vi "Camera Barcode.vi"() -> ()   [LabVIEW 2017]
uses:
  IMAQCV/PIIO/Core/PIIO DIO.ctl
  IMAQCV/GPIO/GPIO Pins.ctl
  <vilib>/Platform/TimedLoop/XDataNode/timing_clust.ctl
  <vilib>/Platform/TimedLoop/XDataNode/nitl_modes.ctl
  <vilib>/Platform/TimedLoop/XDataNode/wakeup.ctl
  <vilib>/vision/Instrument.llb/Barcode Search Options.ctl
  <vilib>/platform/TimedLoop/XDataNode/XDataNode.xnode
  IMAQCV/PIIO.lvlib
  IMAQCV/IMAQCV.lvlib
  IMAQCV/LVOpenCV.lvlib
  <vilib>/Platform/TimedLoop/XDataNode/XDNodeRunTimeDep.lvlib
  <vilib>/vision/NI_Vision_Development_Module.lvlib
panel:
  in  "PIN":T1 items=["L1", "L2"]
  in  "Shutter (us, 0=auto)":i32
  in  "Effect":T2(ring)
  in  "Meter":enum16{"AVERAGE", "SPOT", "BACKLIT", "MATRIX"}(ring)
  in  "AWB":T3(ring)
  in  "Flip Vertical":bool
  in  "Flip Horizontal":bool
  in  "Rotation":u16(ring) items=["0", "90", "180", "270"]
  in  "Sharpness":i32(slide)=50 scale=0.0..100.0
  in  "Saturation":i32(slide)=50 scale=0.0..100.0
  in  "Contrast":i32(slide)=50 scale=0.0..100.0
  in  "Brightness":i32(slide)=50 scale=0.0..100.0
  in  "Gain (0=auto)":i32(slide) scale=0.0..100.0
  in  "LED Control":bool
  in  "FPS":i32=90
  in  "RGB LED 8x8":u32[][](array[colorbox])=[[0, 0, 16777215, 16777215, 16777215, 16777215, 16777215, 16777215], [0, 16777215, 16777215, 16777215, 16777215, 16777215, 16777215, 16777215], [16777215, 16777215, 16777215, 16777215, 16777215, 16777215, 16777215, 16777215], [16777215, 16777215, 0, 0, 0, 0, 0, 0], [16777215, 16777215, 0, 0, 0, 0, 0, 0], [16777215, 16777215, 0, 0, 0, 0, 0, 0], [16777215, 16777215, 0, 0, 0, 0, 0, 0], [0, 16777215, 16777215, 16777215, 16777215, 0, 0, 0]]
  out "picture":picture
  in  "Image Size":T4(ring)=enum."640 (H)   x  480 (V) "
  in  "LED Flash":bool
  out "moving speed (ms)":u32
  out "barcode process time (ms)":u32
  out "Barcode ANSI/CEN/ISO Grading Report":T5(array[cluster])
  out "Barcode Read":cluster{"Data":string, "Barcode Type":string}[](array[cluster])
  out "Number of Barcodes Found":u32
  in  "delay (ms)":u32=150
  out "DI-CH4":bool
  out "DI-CH3":bool
  out "DI-CH2":bool
  out "DI-CH1":bool
  in  "stop":bool
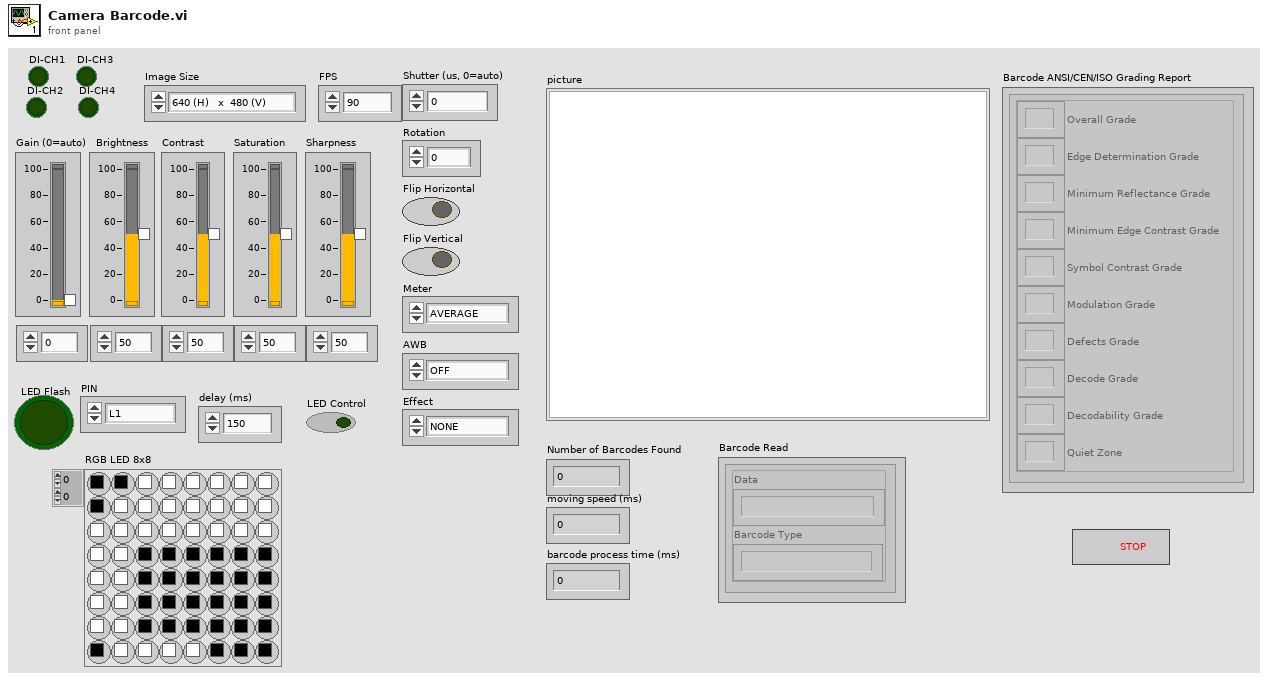
[diagram p1: front panel]
types:
  T1 = typedef "PIIO.lvlib/PIIO DIO.ctl" = u8
  T2 = enum16{"NONE", "NEGATIVE", "SOLARIZE", "SKETCH", "DENOISE", "EMBOSS", "OILPAINT", "HATCH", "GPEN", "PASTEL", "WATERCOLOR", "FILM", "BLUR", "SATURATION", "COLORSWAP", "WASHEDOUT", "POSTERISE", "COLORPOINT", "COLORBALANCE", "CARTOON"}
  T3 = enum16{"OFF", "AUTO", "SUNLIGHT", "CLOUDY", "SHADE", "TUNGSTEN", "FLUORESCENT", "INCANDESCENT", "FLASH"}
  T4 = enum16{"320 (H)   x  240 (V)", "352(H)    x  288 (V)", "640 (H)   x  480 (V) ", "800 (H)   x  600 (V)", "1024 (H) x  768 (V)", "1280 (H) x  720 (V)", "1280 (H) x  960 (V)", "1280 (H) x 1024 (V)", "1920 (H) x 1080 (V)"}
  T5 = cluster{"Overall Grade":string, "Edge Determination Grade":string, "Minimum Reflectance Grade":string, "Minimum Edge Contrast Grade":string, "Symbol Contrast Grade":string, "Modulation Grade":string, "Defects Grade":string, "Decode Grade":string, "Decodability Grade":string, "Quiet Zone":string}[]
  T6 = typedef "PIIO.lvlib/GPIO Pins.ctl" = u8
  T7 = cluster{"GPIO":T6[], "MODE":enum8{"INPUT", "OUTPUT"}[]}
  T8 = typedef "Image Type" = u32
  T9 = typedef "IMAQCV.lvlib/IMAQCV Image.ctl" = refnum<vi>
  T10 = typedef "IMAQ Image.ctl" = refnum<image>
  T11 = typedef "XDNodeRunTimeDep.lvlib/timing_clust.ctl" = cluster{"Expected End [f-1]":u64, "Actual End [f-1]":u64, "Finished Late? [f-1]":bool, "Expected End [i-1]":u64, "Actual End [i-1]":u64, "Finished Late? [i-1]":bool, "Expected Start [i]":u64, "Actual Start [i]":u64, "Expected Start [f]":u64, "Actual Start [f]":u64, "Source Name":string, "Structure Name":string, "Period":i64, "Deadline":i64, "Offset":i64, "Start":i64, "Priority":i32, "Timeout":i32, "Mode":T12, "Wakeup Reason":T13, "Error":errorcluster, "Source Type":string, "Secondary Source Type":string, "Global End Time":u64, "Global Start Time":u64, "Frame Duration":u64, "Iteration Duration":u64, "Assigned CPU":i32, "I/O Scan Engine Mode":u32}
  T12 = typedef "XDNodeRunTimeDep.lvlib/nitl_modes.ctl" = enum32{"No Change", "Process missed periods, maintain original phase", "Discard missed periods, maintain original phase", "Process missed periods, ignore original phase", "Discard missed periods, ignore original phase"}
  T13 = typedef "XDNodeRunTimeDep.lvlib/wakeup.ctl" = enum32{"Normal", "Aborted", "Asynchronous wakeup", "Timing source error", "Timed loop error", "Timeout"}
  T14 = typedef "Barcode Search Options.ctl" = cluster{"Min Bar Width":u32, "Min Edge Strength":u32, "Min Bars":u32, "Skip Location Search?":bool}
  T15 = cluster{"Calculate Grading Report":bool, "Scan Width ":i32}
  T16 = cluster{"Data":string, "Special Char 1":string, "Special Char 2":string, "Checksum(s)":string, "Barcode Type":u32, "Confidence Level":sgl, "Bounding Box":cluster{"x":sgl, "y":sgl}[]}[]
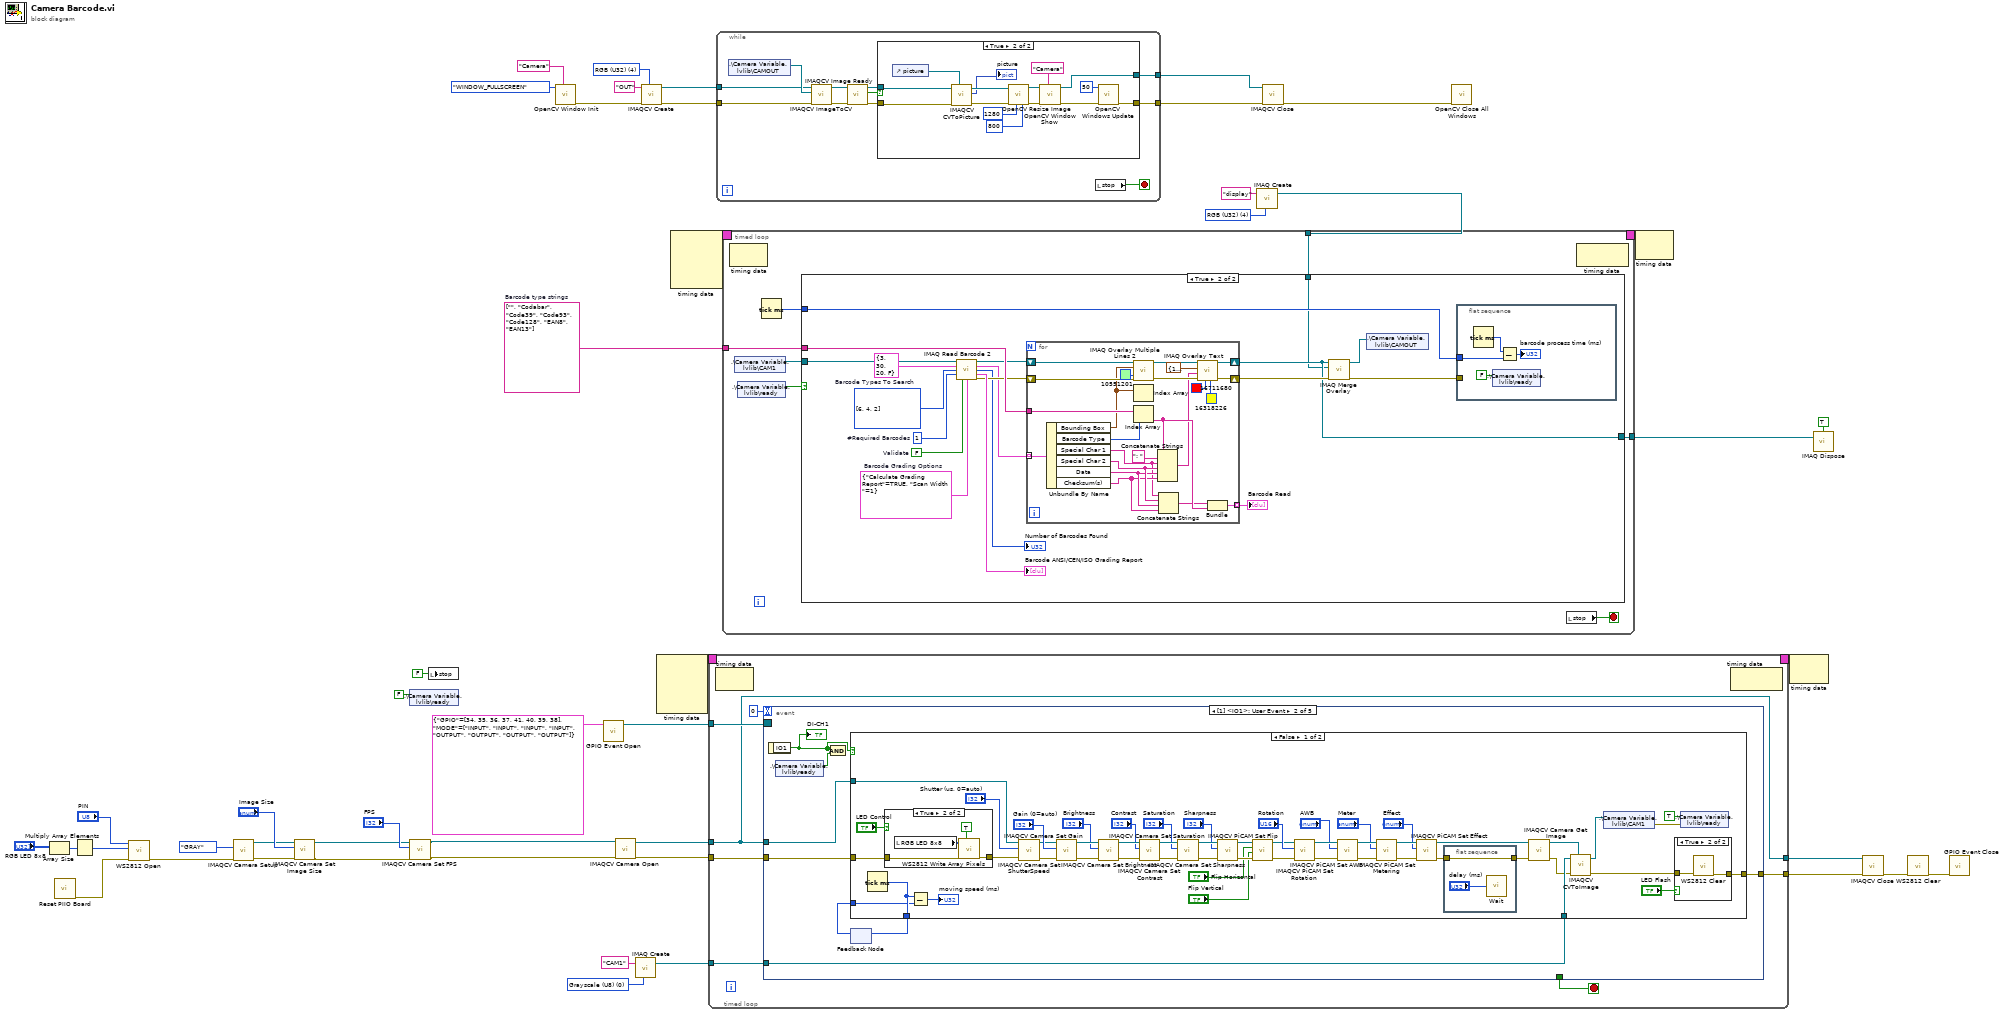
[diagram p0: block diagram]
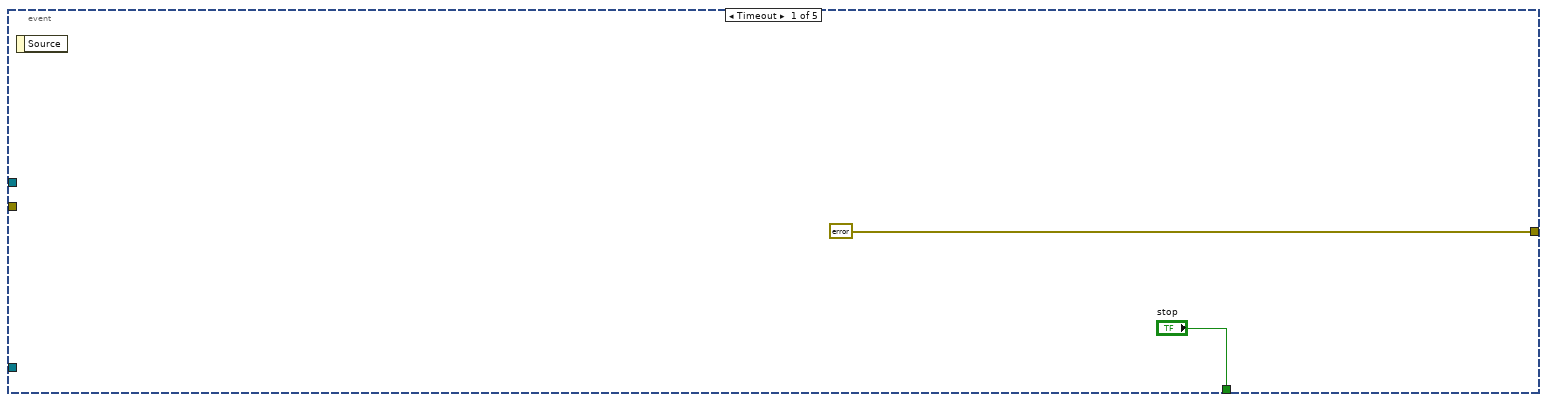
[diagram p4: hidden frame]
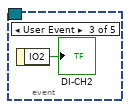
[diagram p8: hidden frame]
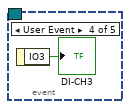
[diagram p9: hidden frame]
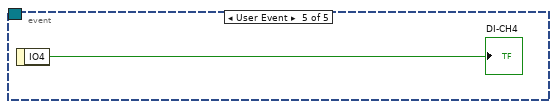
[diagram p10: hidden frame]
diagram:
  w19 = T8 4 items=["Grayscale (U8)", "Grayscale (I16)", "Grayscale (SGL)", "Complex (CSG)", "RGB (U32)", "HSL (U32)", "RGB (U64)", "Grayscale (U16)"] ("Image Type")
  w33 = string[] ["", "Codabar", "Code39", "Code93", "Code128", "EAN8", "EAN13"]  # Barcode type strings
  w38 = u32 4 items=["Grayscale (U8)", "Grayscale (I16)", "Grayscale (SGL)", "Complex (CSG)", "RGB (U32)", "HSL (U32)", "RGB (U64)", "Grayscale (U16)"] ("Image Type")
  w43 = T8 0 items=["Grayscale (U8)", "Grayscale (I16)", "Grayscale (SGL)", "Complex (CSG)", "RGB (U32)", "HSL (U32)", "RGB (U64)", "Grayscale (U16)"] ("Image Type")
  n1 = Array Size(array="RGB LED 8x8") -> (size(s)=w9:i32[])
  n2 = call "Reset PIIO Board.vi"() -> ("error out"=w10:errorcluster)  [unwired: 11 in]
  n3 = Multiply Array Elements(1:w9) -> (0:w7:i32)
  n4 = call "WS2812 Open.vi"("Error In"=w10, "Number of LEDs"=w7, "PIN"="PIN") -> ("Error Out"=w27:errorcluster)  [unwired: 8 in]
  n5 = call "IMAQCV Camera Setup.vi"("error in (no error)"=w27, "type"=enum16{"GRAY", "COLOR"}."GRAY") -> ("error out"=w28:errorcluster, "image out"=w29:T9)  [unwired: 8 in]
  n6 = call "IMAQCV Camera Set Image Size.vi"("error in (no error)"=w28, "Image Size"="Image Size", "image in"=w29) -> ("error out"=w6:errorcluster, "image out"=w5:T9)  [unwired: 7 in]
  n7 = shared-variable ".\\Camera Variable.lvlib\\ready"(FALSE ("outReady")) -> ()  [unwired: 1 in, 1 out]
  n8 = call "IMAQCV Camera Set FPS.vi"("error in (no error)"=w6, "FPS"="FPS", "image in"=w5) -> ("error out"=w4:errorcluster, "image out"=w3:T9)  [unwired: 7 in]
  n9 = local write "stop"(FALSE ("stop")) -> ()
  n10 = call "OpenCV Window Init.vi"("window name"="Camera", "mode"=enum8{"WINDOW_AUTOSIZE", "WINDOW_FULLSCREEN"}."WINDOW_FULLSCREEN") -> ("error out"=w15:errorcluster)  [unwired: 9 in]
  n11 = call "GPIO Event Open.vi"("GPIO"=T7 {"GPIO"=[34, 35, 36, 37, 41, 40, 39, 38], "MODE"=[enum."INPUT", enum."INPUT", enum."INPUT", enum."INPUT", enum."OUTPUT", enum."OUTPUT", enum."OUTPUT", enum."OUTPUT"]}) -> ("Event Registration Refnum"=w11:refnum<event-registration>)  [unwired: 9 in, 1 out]
  n12 = call "IMAQCV Camera Open.vi"("error in (no error)"=w4, "image in"=w3) -> ("error out"=w14:errorcluster, "image out"=w13:T9)  [unwired: 8 in]
  n13 = call "IMAQ Create"("Image Name"="CAM1", "Image Type"=w43) -> ("New Image"=w42:T10)  [unwired: 3 in, 1 out]
  n14 = call "IMAQCV Create.vi"("Image Type"=w38, "error in (no error)"=w15, "Image Name"="OUT") -> ("error out"=w16:errorcluster, "Image Out"=w18:T9)  [unwired: 7 in]
  n15 = node-c288() -> (w35:T11)  [unwired: 4 in]
  n16 = node-c288() -> (w26:T11)  [unwired: 4 in]
  n17 = timed-loop {
    tunnel: w11 -> [w53]
    tunnel: [w52] -> w47
    tunnel: w14 -> [w51]
    tunnel: w13 -> [w50]
    tunnel: [w50] -> w45
    tunnel: w42 -> [w49]
    timing: w35 -> [_]
    timing-out: [_] -> w34
    stop <- w55 stop-if-true
    n18 = node-c288() -> ()  [unwired: 1 in, 1 out]
    n19 = event shown="[1] <IO1>: User Event" {
      selector: w53 -> [_ _ _ _ _]
      dyn-events: _ -> [_ _ _ _ _]
      timeout: 0 -> [_ _ _ _ _]
      tunnel: ["stop" _ _ _ _] -> w55
      tunnel: [errorcluster {"status"=FALSE, "code"=0, "source"=""} ("error out") w66 _ _ _] -> w52
      tunnel: w50 -> [_ w65 _ _ _]
      tunnel: w51 -> [_ w67 _ _ _]
      tunnel: w49 -> [_ w64 _ _ _]
      event Timeout {
        n20 = event-data() -> ()  [unwired: 1 in, 1 out]
      }
      event User Event {
        n21 = event-data() -> ("IO1"=w60:bool)  [unwired: 1 in]
        "DI-CH1" <- w60
        n22 = shared-variable ".\\Camera Variable.lvlib\\ready"() -> (w61:bool)  [unwired: 1 in, 1 out]
        n23 = And(x=w60, y=w61) -> ()  [unwired: 1 out]
        n24 = feedback #1() -> (w62:u32)  [unwired: 1 in]
        n25 = case shown="False" w60 {
          tunnel: w67 -> [w105 w130]
          tunnel: [w117 w130] -> w66
          tunnel: w65 -> [w69 _]
          tunnel: w64 -> [w108 _]
          tunnel: w62 -> [w112 w129]
          tunnel: [w113 w129] -> w63
          frame False {
            n26 = Tick Count (ms)() -> (millisecond timer value=w113:u32)
            n27 = case shown="True" "LED Control" {
              tunnel: w105 -> [w119 w123]
              tunnel: [w119 w120] -> w71
              frame False {
              }
              frame True {
                n28 = local read "RGB LED 8x8"() -> (w121:u32[][])
                n29 = call "WS2812 Write Array Pixels.vi"("Refresh? (True)"=TRUE, "Error In"=w123, "pixmap"=w121) -> ("Error Out"=w120:errorcluster)  [unwired: 8 in]
              }
            }
            n30 = Subtract(x=w113, y=w112) -> (x-y=→"moving speed (ms)":u32)
            n31 = call "IMAQCV Camera Set ShutterSpeed.vi"("error in (no error)"=w71, "shutter speed (us, 0=auto)"="Shutter (us, 0=auto)", "image in"=w69) -> ("error out"=w74:errorcluster, "image out"=w73:T9)  [unwired: 7 in]
            n32 = call "IMAQCV Camera Set Gain.vi"("error in (no error)"=w74, "gain (0=auto)"="Gain (0=auto)", "image in"=w73) -> ("error out"=w102:errorcluster, "image out"=w103:T9)  [unwired: 7 in]
            n33 = call "IMAQCV Camera Set Brightness.vi"("error in (no error)"=w102, "brightness"="Brightness", "image in"=w103) -> ("error out"=w101:errorcluster, "image out"=w98:T9)  [unwired: 7 in]
            n34 = call "IMAQCV Camera Set Contrast.vi"("error in (no error)"=w101, "contrast"="Contrast", "image in"=w98) -> ("error out"=w100:errorcluster, "image out"=w97:T9)  [unwired: 7 in]
            n35 = call "IMAQCV Camera Set Saturation.vi"("error in (no error)"=w100, "saturation"="Saturation", "image in"=w97) -> ("error out"=w99:errorcluster, "image out"=w96:T9)  [unwired: 7 in]
            n36 = call "IMAQCV Camera Set Sharpness.vi"("error in (no error)"=w99, "sharpness"="Sharpness", "image in"=w96) -> ("error out"=w89:errorcluster, "image out"=w88:T9)  [unwired: 7 in]
            n37 = call "IMAQCV PiCAM Set Flip.vi"("error in (no error)"=w89, "vertical"="Flip Vertical", "horizontal"="Flip Horizontal", "image in"=w88) -> ("error out"=w87:errorcluster, "image out"=w86:T9)  [unwired: 6 in]
            n38 = call "IMAQCV PiCAM Set Rotation.vi"("error in (no error)"=w87, "Rotation"="Rotation", "image in"=w86) -> ("error out"=w83:errorcluster, "image out"=w82:T9)  [unwired: 7 in]
            n39 = call "IMAQCV PiCAM Set AWB.vi"("error in (no error)"=w83, "AWB"="AWB", "image in"=w82) -> ("error out"=w80:errorcluster, "image out"=w78:T9)  [unwired: 7 in]
            n40 = call "IMAQCV PiCAM Set Metering.vi"("error in (no error)"=w80, "mode"="Meter", "image in"=w78) -> ("error out"=w79:errorcluster, "image out"=w77:T9)  [unwired: 7 in]
            n41 = call "IMAQCV PiCAM Set Effect.vi"("error in (no error)"=w79, "effect"="Effect", "image in"=w77) -> ("error out"=w70:errorcluster, "image out"=w68:T9)  [unwired: 7 in]
            n42 = flat-sequence {
              tunnel: [w127] -> w118
              tunnel: w70 -> [w127]
              frame #0 {
                n43 = call "Wait"("Count(mSec)"="delay (ms)") -> ()  [unwired: 1 out]
              }
            }
            n44 = call "IMAQCV Camera Get Image.vi"("error in (no error)"=w118, "image in"=w68) -> ("error out"=w107:errorcluster, "image out"=w106:T9)  [unwired: 8 in]
            n45 = call "IMAQCV CVToImage.vi"("cvimage in"=w106, "error in (no error)"=w107, "Variant In"=w108) -> ("error out"=w114:errorcluster, "Variant Out"=w109:refnum<image>)  [unwired: 7 in]
            n46 = shared-variable ".\\Camera Variable.lvlib\\CAM1"(w109) -> (error out=w115:errorcluster)  [unwired: 1 in]
            n47 = case shown="True" "LED Flash" {
              tunnel: [w124 w126] -> w117
              tunnel: w114 -> [w124 w125]
              frame False {
              }
              frame True {
                n48 = call "WS2812 Clear.vi"("Error In"=w125) -> ("Error Out"=w126:errorcluster)  [unwired: 10 in]
              }
            }
            n49 = shared-variable ".\\Camera Variable.lvlib\\ready"(TRUE ("ready"), error in=w115) -> ()  [unwired: 1 out]
          }
          frame True {
          }
        }
        n50 = feedback-in #1(w63) -> ()
      }
      event User Event {
        n51 = event-data() -> ("IO2"=→"DI-CH2":bool)  [unwired: 1 in]
      }
      event User Event {
        n52 = event-data() -> ("IO3"=→"DI-CH3":bool)  [unwired: 1 in]
      }
      event User Event {
        n53 = event-data() -> ("IO4"=→"DI-CH4":bool)  [unwired: 1 in]
      }
    }
    n54 = node-c288() -> ()  [unwired: 1 in, 1 out]
  }
  n55 = while {
    tunnel: [w143] -> w24
    tunnel: [w142] -> w23
    tunnel: w18 -> [w137]
    tunnel: w16 -> [w134]
    stop <- w144 stop-if-true
    n56 = shared-variable ".\\Camera Variable.lvlib\\CAMOUT"() -> (w138:refnum<image>)  [unwired: 1 in, 1 out]
    n57 = call "IMAQCV ImageToCV.vi"("error in (no error)"=w134, "Variant In"=w138, "CV in"=w137) -> ("error out"=w135:errorcluster, "CV out"=w136:T9)  [unwired: 7 in]
    n58 = call "IMAQCV Image Ready.vi"("error in (no error)"=w135, "image in"=w136) -> ("error out"=w140:errorcluster, "ready?"=w139:bool, "image out"=w141:T9)  [unwired: 7 in]
    n59 = case shown="True" w139 {
      tunnel: [w145 w158] -> w143
      tunnel: [w146 w157] -> w142
      tunnel: w141 -> [w145 w149]
      tunnel: w140 -> [w146 w150]
      frame False {
      }
      frame True {
        n60 = control-ref of="picture"() -> (w148:refnum<vi>)
        n61 = call "IMAQCV CVToPicture.vi"("picture ref"=w148, "error in (no error)"=w150, "image"=w149) -> ("error out"=w151:errorcluster, "picture"=→"picture":picture, "image out"=w152:T9)  [unwired: 6 in]
        n62 = call "OpenCV Resize Image.vi"("height"=u32 800, "width"=u32 1280, "error in (no error)"=w151, "image in"=w152) -> ("error out"=w153:errorcluster, "image out"=w154:T9)  [unwired: 6 in]
        n63 = call "OpenCV Window Show.vi"("window name"="Camera", "error in (no error)"=w153, "image in"=w154) -> ("error out"=w159:errorcluster, "image out"=w158:T9)  [unwired: 7 in]
        n64 = call "OpenCV Windows Update.vi"("error in (no error)"=w159, "wait ms"=50) -> ("error out"=w157:errorcluster)  [unwired: 8 in, 1 out]
      }
    }
    n65 = local read "stop"() -> (w144:bool)
  }
  n66 = call "IMAQ Create"("Image Name"="display", "Image Type"=w19) -> ("New Image"=w17:T10)  [unwired: 3 in, 1 out]
  n67 = timed-loop {
    tunnel: w33 -> [w167]
    timing: w26 -> [_]
    timing-out: [_] -> w25
    tunnel: [w163] -> w22
    tunnel: w17 -> [w162]
    stop <- w168 stop-if-true
    n68 = node-c288() -> ()  [unwired: 1 in, 1 out]
    n69 = shared-variable ".\\Camera Variable.lvlib\\CAM1"() -> (w165:refnum<image>)  [unwired: 1 in, 1 out]
    n70 = shared-variable ".\\Camera Variable.lvlib\\ready"() -> (w164:bool)  [unwired: 1 in, 1 out]
    n71 = Tick Count (ms)() -> (millisecond timer value=w166:u32)
    n72 = case shown="True" w164 {
      tunnel: w167 -> [_ w190]
      tunnel: w166 -> [_ w189]
      tunnel: w165 -> [w171 w187]
      tunnel: [w171 w186] -> w163
      tunnel: w162 -> [_ w185]
      frame False {
      }
      frame True {
        w175 = T15 {"Calculate Grading Report"=TRUE, "Scan Width "=1}  # Barcode Grading Options
        w177 = u32 1  # #Required Barcodes
        w178 = u32[] [6, 4, 2] items=["Reserved", "Codabar", "Code 39", "Code 93", "Code 128", "EAN 8", "EAN 13", "Interleaved 2 of 5", "MSI", "UPCA", "Pharmacode", "RSS Limited"]  # Barcode Types To Search
        w176 = FALSE  # Validate
        n73 = call "IMAQ Read Barcode 2"("Image"=w187, "Barcode Search Options"=T14 {"Min Bar Width"=3, "Min Edge Strength"=30, "Min Bars"=20, "Skip Location Search?"=FALSE}, "Barcode Types To Search"=w178, "Num of Required Barcodes"=w177, "Validate"=w176, "Barcode Grading Options"=w175) -> ("Image (duplicate)"=w180:T10, "Barcodes"=w179:T16, "Num of Barcodes"=→"Number of Barcodes Found":u32, "Barcode ANSI/CEN/ISO Grading Report"=→"Barcode ANSI/CEN/ISO Grading Report":T5, "error out"=w181:errorcluster)  [unwired: 5 in]
        n74 = for {
          tunnel: w179 -> [w213] mode=indexing
          tunnel: w190 -> [w212]
          shift-right: [w208] -> w186
          shift-left: w180 -> [w204]
          shift-right: [w205] -> w188
          shift-left: w181 -> [w207]
          tunnel: [w201] -> w172 mode=indexing
          n75 = Unbundle By Name(w213) -> ("Bounding Box"=w203:cluster{"x":sgl, "y":sgl}[], "Barcode Type"=w202:u32, "Special Char 1"=w194:string, "Special Char 2"=w198:string, "Data"=w197:string, "Checksum(s)"=w196:string)
          n76 = call "IMAQ Overlay Multiple Lines 2"("Image"=w204, "Line End Points"=w203, "Color"=u32 10551201, "error in (no error)"=w207) -> ("Image Out"=w210:T10, "error out"=w206:errorcluster)  [unwired: 10 in]
          n77 = Index Array(array=w203) -> ()  [unwired: 1 in, 1 out]
          n78 = Index Array(array=w212, index=w202) -> (element=w200:string)
          n79 = Concatenate Strings(w200, ": " ("string"), w194, w198, w197, w196) -> (w199:string)
          n80 = Concatenate Strings(w194, w198, w197, w196) -> (w195:string)
          n81 = call "IMAQ Overlay Text"("BG Color (Transparent)"=u32 16318226, "Text Color (black)"=u32 16711680, "error in (no error)"=w206, "String"=w199, "Origin"=cluster{"X":i32, "Y":i32} {"X"=10, "Y"=20}, "Image"=w210) -> ("error out"=w205:errorcluster, "Image Out"=w208:T10)  [unwired: 4 in]
          n82 = Bundle(w195, w200) -> (w201:cluster{string, string})  [unwired: 1 in]
        }
        "Barcode Read" <- w172
        n83 = call "IMAQ Merge Overlay"("error in (no error)"=w188, "Image Dst"=w185, "Image Src"=w186) -> ("error out"=w183:errorcluster, "Image Dst Out"=w184:T10)  [unwired: 7 in]
        n84 = shared-variable ".\\Camera Variable.lvlib\\CAMOUT"(w184) -> ()  [unwired: 1 in, 1 out]
        n85 = flat-sequence {
          tunnel: w189 -> [w216]
          tunnel: w183 -> [_]
          frame #0 {
            n86 = Tick Count (ms)() -> (millisecond timer value=w217:u32)
            n87 = shared-variable ".\\Camera Variable.lvlib\\ready"(FALSE ("outReady")) -> ()  [unwired: 1 in, 1 out]
            n88 = Subtract(x=w217, y=w216) -> (x-y=→"barcode process time (ms)":u32)
          }
        }
      }
    }
    n89 = local read "stop"() -> (w168:bool)
    n90 = node-c288() -> ()  [unwired: 1 in, 1 out]
  }
  n91 = call "IMAQCV Close.vi"("error in (no error)"=w23, "Image"=w24) -> ("error out"=w40:errorcluster)  [unwired: 9 in]
  n92 = call "OpenCV Close All Windows.vi"("error in (no error)"=w40) -> ()  [unwired: 10 in, 1 out]
  n93 = node-c288(w25) -> ()  [unwired: 1 out]
  n94 = node-c288(w34) -> ()  [unwired: 1 out]
  n95 = call "IMAQ Dispose"("All Images? (No)"=TRUE, "Image"=w22) -> ()  [unwired: 4 in, 1 out]
  n96 = call "IMAQCV Close.vi"("error in (no error)"=w47, "Image"=w45) -> ("error out"=w48:errorcluster)  [unwired: 9 in]
  n97 = call "WS2812 Clear.vi"("Error In"=w48) -> ("Error Out"=w46:errorcluster)  [unwired: 10 in]
  n98 = call "GPIO Event Close.vi"("error in (no error)"=w46) -> ()  [unwired: 10 in, 1 out]
